vi "Magnetic Control.vi"() -> ()   [LabVIEW 2012]
doc: "I. Description:\nThis example demonstrates how to output multiple Voltage Updates (Samples) to an Analog Output Channel in a software timed loop.\n\nII. Instructions for Running:\n1. Select the Physical Channel to correspond to where your signal is output on the DAQ device.\n2. Enter the Minimum and Maximum Voltage Ranges\nNote: Use the Cont Acq Multiple Samples example to verify you are generating the correct output on the DAQ device.\n3. Set the loop rate.\n4. Run theVI.\n5. Stop the VI when desired.\n\nIII. Block Diagram Steps:\n1. Create an Analog Output Voltage channel.\n2. The Array Data is a sinewave with 1000 points, generates 5 cycles, and has an amplitude of 2.\n3. Call the Start VI\n4. Write one data point from the array (modulo indexed to loop count) until the user hits the stop button or an error occurs. The loop rate is settable to 1 millisecond. \n5. Call the Clear Task VI to clear the Task.\n6. Use the popup dialog box to display an error if any. \n\nIV. I/O Connections Overview:\nMake sure your signal output terminal matches the Physical Channel I/O Control. For further connection information, refer to your hardware reference manual."
uses:
  <vilib>/Utility/error.llb/DialogType.ctl
  <vilib>/ULx/Create Channel.llb/ULx Create Channel (AO-Voltage-Basic).vi
  <vilib>/ULx/Write.llb/ULx Write (Analog 1D DBL NChan 1Samp).vi
panel:
  out "Running":bool
  in  "Exit":bool
  in  "Up Coil Voltage(V)                                        Down Coil Voltage (V)":dbl[](array[numeric])=[0.0, 1.4099999999999995, 1.6, 0.0, 0.0, 1.415, 1.6, 0.0, 4.5]
  in  "Maximum Value":dbl=5.5 format="%0.2f"
  in  "Minimum Value":dbl format="%0.2f"
  in  "Run/Stop":bool caption="stop"
  # "Channel Parameters"
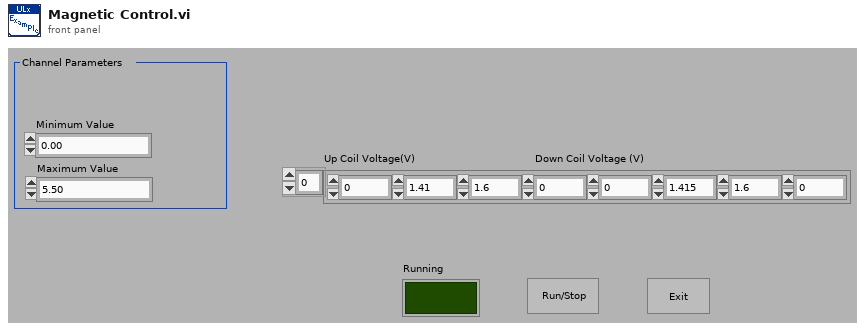
[diagram p1: front panel]
types:
  T1 = typedef "DialogType.ctl" = u16
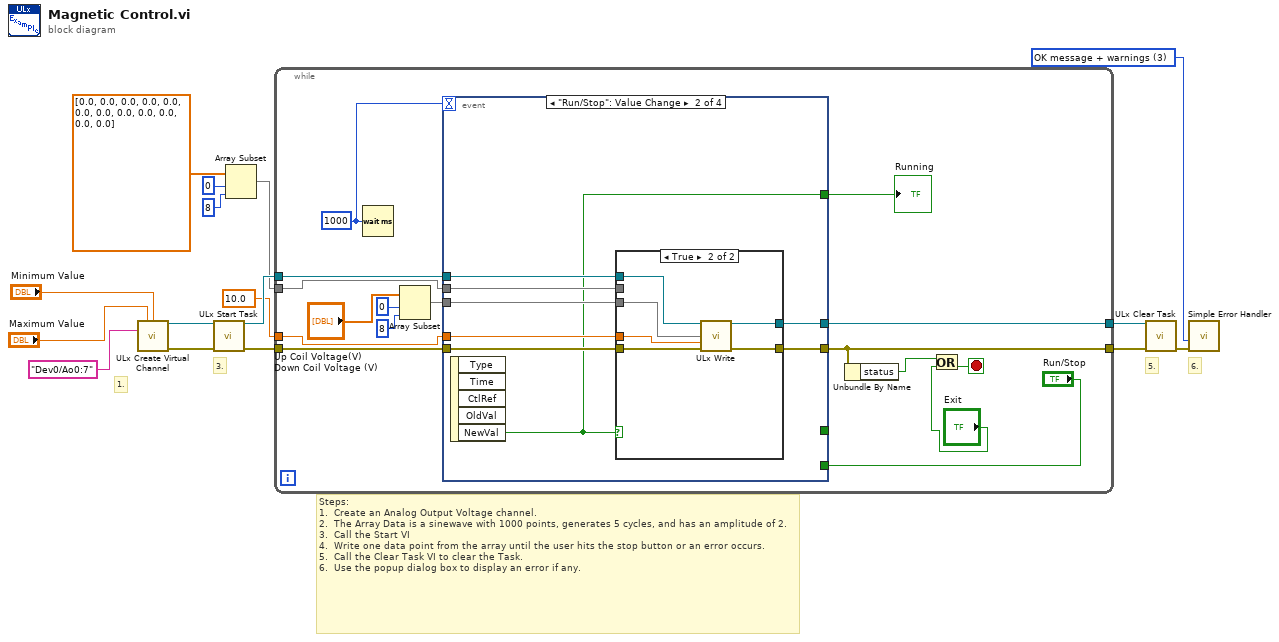
[diagram p0: block diagram]
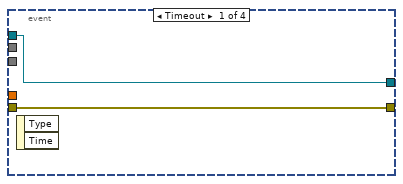
[diagram p2: hidden frame]
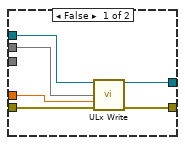
[diagram p3: hidden frame]
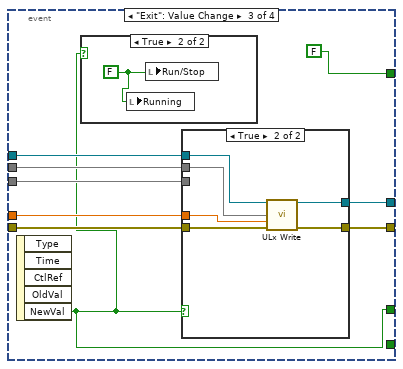
[diagram p4: hidden frame]
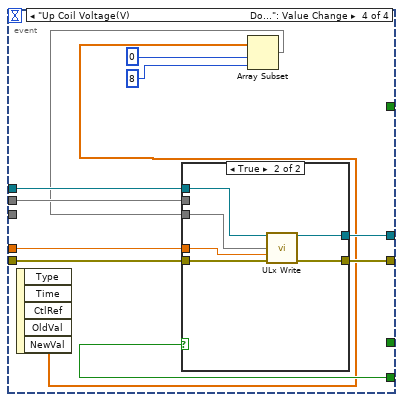
[diagram p7: hidden frame]
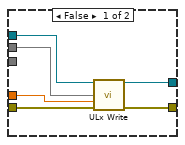
[diagram p8: hidden frame]
diagram:
  w11 = T1 3 items=["no dialog", "OK message", "continue or stop message", "OK message + warnings", "continue/stop + warnings"] ("type of dialog (OK msg:1)")
  # "6."
  # "5."
  # "Steps: \n1.  Create an Analog Output Voltage channel.\n2.  The Array Data is a sinewave with 1000 points, generates 5 cycles, and has an amplitude of 2.\n3.  Call the Start VI\n4.  Write one data point from the array until the user hits the stop button or an error occurs. \n5.  Call the Clear Task VI to clear the Task.\n6.  Use the popup dialog box to display an error if any."
  # "3."
  # "1."
  n1 = call-poly <vilib>:"ULx Create Virtual Channel.vi"("maximum value"="Maximum Value", "minimum value"="Minimum Value", "physical channels"="Dev0/Ao0:7") -> ("task out"=w10:refnum<k24>, "error out"=w9:errorcluster)  [unwired: 11 in]
  n2 = call <vilib>:"ULx Start Task.vi"("task in"=w10, "error in"=w9) -> ("task out"=w12:refnum<k24>, "error out"=w14:errorcluster)  [unwired: 12 in]
  n3 = Array Subset(array=dbl[] [0.0, 0.0, 0.0, 0.0, 0.0, 0.0, 0.0, 0.0, 0.0, 0.0, 0.0, 0.0] ("Voltage(V) 2"), index=0, length=8) -> (w1:dbl[])
  n4 = while {
    tunnel: w14 -> [w31]
    tunnel: w12 -> [w32]
    tunnel: w1 -> [w28]
    tunnel: [w30] -> w7
    tunnel: [w23] -> w6
    tunnel: 10.0 ("timeout") -> [w29]
    stop <- w22 stop-if-true
    w19 = 1000
    n5 = Wait (ms)(milliseconds to wait=w19) -> ()  [unwired: 1 out]
    n6 = Array Subset(array="Up Coil Voltage(V)                                        Down Coil Voltage (V)", index=0, length=8) -> (w24:dbl[])
    n7 = event shown="[1] \"Run/Stop\": Value Change" {
      selector: _ -> [_ _ _ _]
      dyn-events: _ -> [_ _ _ _]
      timeout: w19 -> [_ _ _ _]
      tunnel: w32 -> [w34 w42 w63 w83]
      tunnel: w31 -> [w33 w41 w62 w82]
      tunnel: w29 -> [_ w40 w61 w81]
      tunnel: w24 -> [_ w39 w60 _]
      tunnel: [w34 w38 w59 w80] -> w30
      tunnel: [w33 w37 w58 w79] -> w23
      tunnel: w28 -> [_ w36 w57 w78]
      tunnel: "Run/Stop" -> [_ _ _ w77]
      tunnel: [_ _ w56 _] -> _
      tunnel: [_ w35 FALSE _] -> w17
      event Timeout {
        n8 = event-data() -> ()  [unwired: 1 in, 2 out]
      }
      event "Run/Stop": Value Change {
        n9 = event-data() -> ("NewVal"=w35:bool)  [unwired: 1 in, 4 out]
        n10 = case shown="True" w35 {
          tunnel: w42 -> [w46 w54]
          tunnel: w41 -> [w45 w53]
          tunnel: w40 -> [w47 w52]
          tunnel: w39 -> [_ w51]
          tunnel: [w44 w50] -> w38
          tunnel: [w43 w49] -> w37
          tunnel: w36 -> [w48 _]
          frame False {
            n11 = call-poly <vilib>:"ULx Write.vi"("task in"=w46, "data"=w48, "timeout"=w47, "error in"=w45) -> ("task out"=w44:refnum<k24>, "error out"=w43:errorcluster)  [unwired: 9 in, 1 out]
          }
          frame True {
            n12 = call-poly <vilib>:"ULx Write.vi"("task in"=w54, "data"=w51, "timeout"=w52, "error in"=w53) -> ("task out"=w50:refnum<k24>, "error out"=w49:errorcluster)  [unwired: 9 in, 1 out]
          }
        }
      }
      event "Exit": Value Change {
        n13 = event-data() -> ("NewVal"=w56:bool)  [unwired: 1 in, 4 out]
        n14 = case shown="True" w56 {
          frame False {
          }
          frame True {
            w64 = FALSE
            n15 = local write "Running"(w64) -> ()
            n16 = local write "Run/Stop"(w64) -> ()
          }
        }
        n17 = case shown="True" w56 {
          tunnel: w63 -> [w66 w72]
          tunnel: w62 -> [w65 w71]
          tunnel: w61 -> [_ w70]
          tunnel: w60 -> [_ _]
          tunnel: [w66 w69] -> w59
          tunnel: [w65 w68] -> w58
          tunnel: w57 -> [_ w67]
          frame False {
          }
          frame True {
            n18 = call-poly <vilib>:"ULx Write.vi"("task in"=w72, "data"=w67, "timeout"=w70, "error in"=w71) -> ("task out"=w69:refnum<k24>, "error out"=w68:errorcluster)  [unwired: 9 in, 1 out]
          }
        }
      }
      event "Up Coil Voltage(V)                                        Down Coil Voltage (V)": Value Change {
        n19 = event-data() -> ("NewVal"=w74:dbl[])  [unwired: 1 in, 4 out]
        n20 = Array Subset(array=w74, index=0, length=8) -> (w73:dbl[])
        n21 = case shown="True" w77 {
          tunnel: w83 -> [w87 w95]
          tunnel: w82 -> [w86 w94]
          tunnel: w81 -> [w88 w93]
          tunnel: w73 -> [_ w92]
          tunnel: [w85 w91] -> w80
          tunnel: [w84 w90] -> w79
          tunnel: w78 -> [w89 _]
          frame False {
            n22 = call-poly <vilib>:"ULx Write.vi"("task in"=w87, "data"=w89, "timeout"=w88, "error in"=w86) -> ("task out"=w85:refnum<k24>, "error out"=w84:errorcluster)  [unwired: 9 in, 1 out]
          }
          frame True {
            n23 = call-poly <vilib>:"ULx Write.vi"("task in"=w95, "data"=w92, "timeout"=w93, "error in"=w94) -> ("task out"=w91:refnum<k24>, "error out"=w90:errorcluster)  [unwired: 9 in, 1 out]
          }
        }
      }
    }
    "Running" <- w17
    n24 = Unbundle By Name(w23) -> ("status"=w21:bool)
    n25 = Or(x=w21, y="Exit") -> (x .or. y?=w22:bool)
  }
  n26 = call <vilib>:"ULx Clear Task.vi"("task in"=w7, "error in"=w6) -> ("error out"=w13:errorcluster)  [unwired: 13 in]
  n27 = call <vilib>:"Simple Error Handler.vi"("type of dialog (OK msg:1)"=w11, "error in (no error)"=w13) -> ()  [unwired: 3 in, 5 out]
